vi "prepCI2_res.vi"   [LabVIEW 2013]
uses:
  <vilib>/DAQmx/create/channels.llb/DAQmx Create Channel (CI-Count Edges).vi
  <vilib>/DAQmx/configure/timing.llb/DAQmx Timing (Sample Clock).vi
  <resource>/objmgr/daqmx.rc
types:
  T1 = cluster{"CH1 AI":tag, "CH1 CI":tag, "CH2 AI":tag, "CH2 CI":tag, "AI X":tag, "AI Y":tag, "AO X-Y":tag, "CH1ST":bool, "CH2ST":bool, "Sigcase":i16, "StageS":i32, "StageL":i32, "data dir":path, "Vp":tag, "Ip":tag, "AO CWlaser":tag, "AO VtoP":tag, "shutter":tag, "488":tag, "532":tag, "640":tag, "LT marker":tag, "image OD":u16, "contour OD":u16, "point OD":u16}
  T2 = typedef "LVRectTypeDef.ctl" = cluster{"Left":i16, "Top":i16, "Right":i16, "Bottom":i16}
  T3 = cluster{"Xpixels":i32, "Vxminref":dbl, "Vxmaxref":dbl, "P":dbl, "Ypixels":i32, "Vyminref":dbl, "Vymaxref":dbl, "srate":sgl, "sAOxy":i32, "timeout":dbl, "type":string, "date":string, "time":string, "Colormap":u16, "Drawing Mode":u16, "Scanning Mode":u16, "square pixels":bool, "square matrix":bool, "Xpixels Img":i32, "Vx-min Img":dbl, "VX-max Img":dbl, "Ypixels Img":i32, "Vy-min Img":dbl, "Vy-max Img ":dbl, "Angle Img":dbl, "autoshutter":bool, "finite":bool, "cont":bool, "wavdet":bool, "measpoints":i32, "avpp":i32, "bufferAO":i32, "bufferAI":i32, "CH1":bool, "CH2":bool, "X":bool, "Y":bool, "Ip":bool, "Vp":bool, "starttick":u32, "waveform":path, "Vx-ref":dbl, "Vy-ref":dbl, "refreshrate":dbl, "refreshbuffer":i32, "tt_cycles":i32, "motorref":refnum<k7>, "mirrorswitch":refnum<k7>, "sample mode":i32, "maxbufferAI":i32, "sampletreshold":dbl, "srateAODO":sgl, "bin":sgl, "Pel":sgl, "Angle draw":dbl, "srate Img":sgl, "ROIimg_plotbounds":T2, "auto OD":bool, "ODfilt":u16, "reset AO_DO":bool}
  T4 = cluster{" CI1":refnum<k21>, "E_CI1":errorcluster}
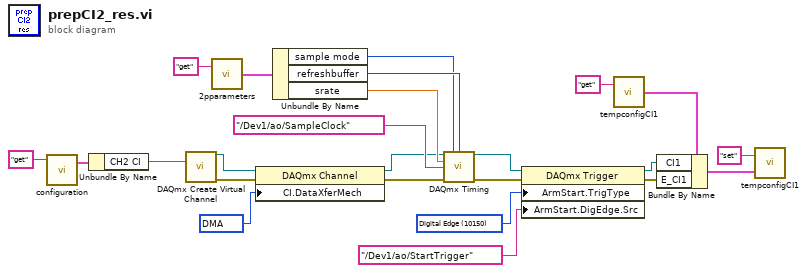
[diagram p0: block diagram]
diagram:
  w3 = 10054 items=["DMA"=10054, "Interrupts"=10204, "Programmed I/O"=10264, "USB Bulk"=12590] ("CI.DataXferMech")
  w23 = 10150 items=["Digital Edge"=10150, "None"=10230] ("ArmStart.TrigType")
  n1 = call "configuration.vi"("command"="get") -> ("config out"=w19:T1)  [unwired: 2 in, 1 out]
  n2 = Unbundle By Name(w19) -> ("CH2 CI"=w18:tag)
  n3 = call-poly <vilib>:"DAQmx Create Virtual Channel.vi"("counter"=w18) -> ("task out"=w21:refnum<k21>, "error out"=w2:errorcluster)  [unwired: 13 in]
  n4 = call "2pparameters.vi"("command"="get") -> ("Params out"=w15:T3)  [unwired: 1 in]
  n5 = property class="DAQmx Channel"(reference=w21, error in=w2, "CI.DataXferMech"=w3) -> (reference out=w4:refnum<k21>, error out=w1:errorcluster)
  n6 = Unbundle By Name(w15) -> ("sample mode"=w5:i32, "refreshbuffer"=w13:i32, "srate"=w6:sgl)
  n7 = call-poly <vilib>:"DAQmx Timing.vi"("task/channels in"=w4, "sample mode"=w5, "samples per channel"=w13, "rate"=w6, "source"=tag "/Dev1/ao/SampleClock", "error in"=w1) -> ("task out"=w16:refnum<k21>, "error out"=w24:errorcluster)  [unwired: 8 in]
  n8 = property class="DAQmx Trigger"(reference=w16, error in=w24, "ArmStart.TrigType"=w23, "ArmStart.DigEdge.Src"=tag "/Dev1/ao/StartTrigger") -> (reference out=w8:refnum<k21>, error out=w7:errorcluster)
  n9 = call "tempconfigCI1.vi"("command"="get") -> ("Temp Config out"=w9:T4)  [unwired: 1 in]
  n10 = Bundle By Name(cluster=w9, "CI1"=w8, "E_CI1"=w7) -> (w12:T4)
  n11 = call "tempconfigCI1.vi"("Temp Config in"=w12, "command"="set") -> ()  [unwired: 1 out]
